vi "Test Dynamic Filter.vi"() -> ()   [LabVIEW 2019]
uses:
  src/Instrument.DAQ/Typedefs/REF.Channel--Cluster.ctl
  src/Instrument.Lockin/Instrument.Lockin.lvclass
  src/Instrument.DAQ/Instrument.DAQ.lvclass
panel:
  out "Array":i32[](array[numeric])
  out "XY Graph 6":cluster{dbl[], dbl[]}[](graph)
  out "XY Graph 4":cluster{dbl[], dbl[]}[](graph)
  out "XY Graph 3":cluster{dbl[], dbl[]}[](graph)
  out "XY Graph 2":cluster{dbl[], dbl[]}[](graph)
  out "XY Graph":cluster{dbl[], dbl[]}[](graph)
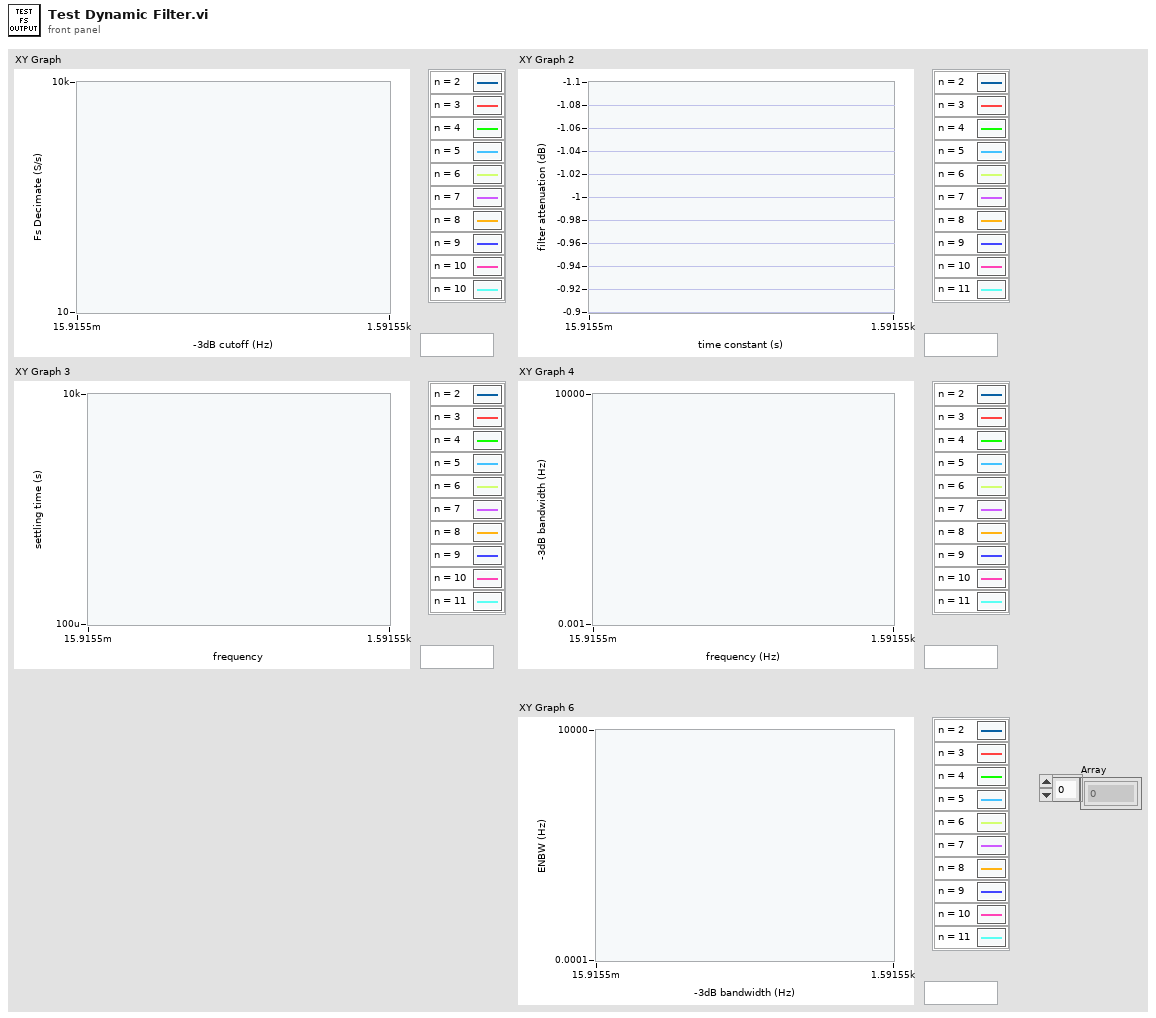
[diagram p1: front panel]
types:
  T1 = typedef "Instrument.Lockin.lvlib/Instrument.DAQ.lvclass/REF.Channel--Cluster.ctl" = cluster{"Enable?":bool, "Channel":i32, "Frequency":dbl, "Phase":dbl, "TC":dbl, "Roll-Off":i32}
  T2 = cluster{"Fs.Output (S/s)":dbl, "Decimation Factor":i32, "Settling Time (s)":dbl, "Noise Bandwidth (Hz)":dbl, "-3dB Bandwidth (Hz)":dbl, "Attenuation (dB)":dbl}
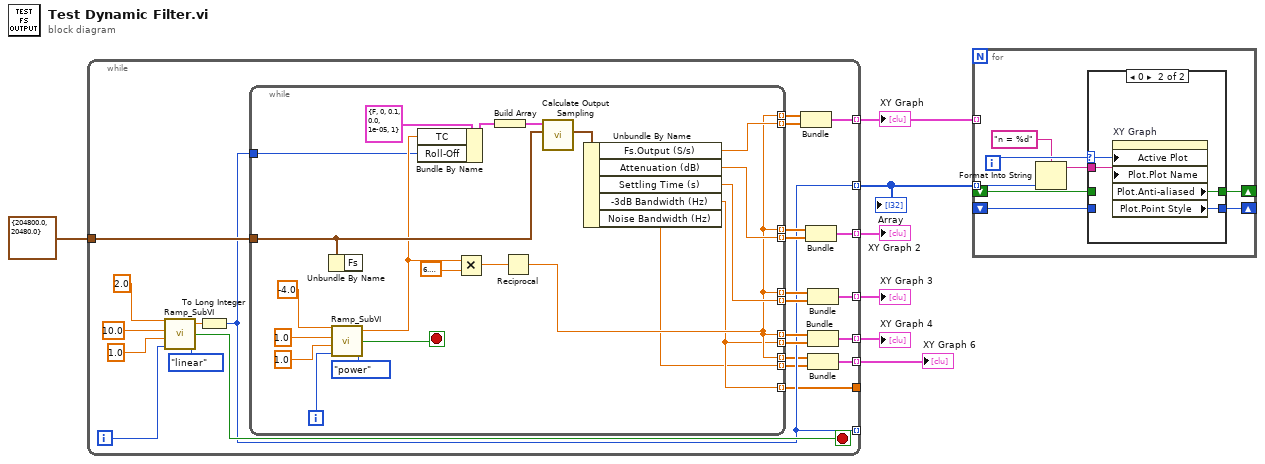
[diagram p0: block diagram]
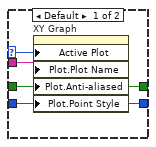
[diagram p2: hidden frame]
diagram:
  n1 = while {
    tunnel: cluster{"Fs":dbl, "#s":dbl} {"Fs"=204800.0, "#s"=20480.0} ("sampling info") -> [w32]
    tunnel: [w30] -> w6 mode=indexing
    tunnel: [w13] -> w5 mode=indexing
    tunnel: [w20] -> w4 mode=indexing
    tunnel: [w15] -> w3 mode=indexing
    tunnel: [w13] -> _ mode=indexing
    tunnel: [w11] -> w2 mode=indexing
    tunnel: [w10] -> w1 mode=indexing
    tunnel: [w8] -> _
    i -> [w23]
    stop <- w24 stop-if-true
    n2 = call <userlib>:"Ramp_SubVI.vi"("Enum"=enum16{"linear", "power"}."linear", "index"=w23, "step"=1.0, "end"=10.0, "start"=2.0) -> ("Stop?"=w24:bool, "Numeric"=w14:dbl)
    n3 = To Long Integer(number=w14) -> (32bit integer=w13:i32)
    n4 = while {
      tunnel: w32 -> [w38]
      tunnel: [w37] -> w31 mode=indexing
      tunnel: [w42] -> w29 mode=indexing
      tunnel: w13 -> [w34]
      tunnel: [w43] -> w22 mode=indexing
      tunnel: [w37] -> w21 mode=indexing
      tunnel: [w37] -> w19 mode=indexing
      tunnel: [w37] -> w18 mode=indexing
      tunnel: [w41] -> w17 mode=indexing
      tunnel: [w36] -> w16 mode=indexing
      tunnel: [w33] -> w12 mode=indexing
      tunnel: [w37] -> w9 mode=indexing
      tunnel: [w36] -> w8 mode=indexing
      i -> [w53]
      stop <- w48 stop-if-true
      n5 = Unbundle By Name(w38) -> ()  [unwired: 1 out]
      n6 = call <userlib>:"Ramp_SubVI.vi"("Enum"=enum16{"linear", "power"}."power", "index"=w53, "step"=1.0, "end"=1.0, "start"=-4.0) -> ("Stop?"=w48:bool, "Numeric"=w35:dbl)
      n7 = Bundle By Name(cluster=T1 {"Enable?"=FALSE, "Channel"=0, "Frequency"=0.1, "Phase"=0.0, "TC"=1e-05, "Roll-Off"=1} ("REF"), "TC"=w35, "Roll-Off"=w34) -> (w46:T1)
      n8 = Multiply(x=w35, y=6.283185307179586) -> (x*y=w39:dbl)
      n9 = Build Array(w46) -> (w45:T1[])
      n10 = Reciprocal(x=w39) -> (1/x=w37:dbl)
      n11 = call "Calculate Output Sampling.vi"("sampling info"=w38, "Cfg_REF"=w45) -> ("Filter Parameters"=w44:T2)  [unwired: 8 in, 1 out]
      n12 = Unbundle By Name(w44) -> ("Fs.Output (S/s)"=w42:dbl, "Attenuation (dB)"=w43:dbl, "Settling Time (s)"=w41:dbl, "-3dB Bandwidth (Hz)"=w36:dbl, "Noise Bandwidth (Hz)"=w33:dbl)
    }
    n13 = Bundle(w31, w29) -> (w30:cluster{dbl[], dbl[]})  [unwired: 1 in]
    n14 = Bundle(w21, w22) -> (w20:cluster{dbl[], dbl[]})  [unwired: 1 in]
    n15 = Bundle(w19, w17) -> (w15:cluster{dbl[], dbl[]})  [unwired: 1 in]
    n16 = Bundle(w18, w16) -> (w11:cluster{dbl[], dbl[]})  [unwired: 1 in]
    n17 = Bundle(w9, w12) -> (w10:cluster{dbl[], dbl[]})  [unwired: 1 in]
  }
  "XY Graph" <- w6
  "XY Graph 2" <- w4
  "XY Graph 3" <- w3
  "XY Graph 4" <- w2
  "XY Graph 6" <- w1
  "Array" <- w5
  n18 = for {
    tunnel: w6 -> [_] mode=indexing
    tunnel: w5 -> [w60] mode=indexing
    shift-right: [w57] -> _
    shift-left: _ -> [w55]
    shift-right: [w56] -> _
    shift-left: _ -> [w54]
    i -> [w61]
    n19 = Format Into String(format string="n = %d", w60) -> (resulting string=w58:string)  [unwired: 2 in, 1 out]
    n20 = case shown="0" w61 {
      selector: w61 -> [w65 w69]
      tunnel: w58 -> [w64 w68]
      tunnel: [w63 w67] -> w57
      tunnel: [w62 w66] -> w56
      tunnel: w55 -> [w63 _]
      tunnel: w54 -> [w62 _]
      frame Default {
        n21 = property on="XY Graph" class="XYGraph (strict)"("Active Plot"=w65, "Plot.Plot Name"=w64, "Plot.Anti-aliased"=w63, "Plot.Point Style"=w62) -> ()  [unwired: 2 in, 2 out]
      }
      frame 0 {
        n22 = property on="XY Graph" class="XYGraph (strict)"("Active Plot"=w69, "Plot.Plot Name"=w68) -> ("Plot.Anti-aliased"=w67:bool, "Plot.Point Style"=w66:u8)  [unwired: 2 in, 2 out]
      }
    }
  }
